vi "main.vi"() -> ()   [LabVIEW 2020]
uses:
  <vilib>/express/express signal manip/GetorSetDDTAttributes/Shared VIs/TimeType.ctl
  5948bca3-3d14-40bf-9fbb-2ba5c3eee3bd.vi
  <vilib>/Analysis/baseanly.llb/Mean (DBL).vi
  faa81322-6883-41b3-8229-1eb533283c0b.vi
  <extravilib>/ChannelInstances/Tag-bool/Read With Abort.vi
  <extravilib>/ChannelInstances/Tag-bool/Write With Abort.vi
  <extravilib>/ChannelInstances/Tag-bool/Instantiate.vi
  <extravilib>/ChannelInstances/Tag-bool/EndpointRead.vi
  <vilib>/express/express signal manip/GetorSetDDTAttributes/Shared VIs/TimeMode Enum to Boolean.vi
  <vilib>/express/express shared/transition.llb/Dynamic To Waveform Array.vi
  <vilib>/express/express signal manip/GetorSetDDTAttributes/Set DDT Attributes/SetT0.vi
  <vilib>/express/express shared/transition.llb/Waveform Array To Dynamic.vi
  <extravilib>/ChannelInstances/Tag-bool/Endpoint.vi
  <vilib>/express/express signal manip/GetorSetDDTAttributes/Set DDT Attributes/Set DDT Properties.xnode
  <extravilib>/ChannelInstances/Tag-bool.lvlib
  <vilib>/ptbypt/NI_PtbyPt.lvlib
  <vilib>/Analysis/NI_AALBase.lvlib
  <vilib>/express/express signal manip/GetorSetDDTAttributes/Shared VIs/GetSetShared.lvlib
panel:
  out "dt":dbl
  in  "?":T1(tab)
  in  "Test Knob":dbl(knob) scale=0.0..10.0
  out "Signal Frequency\n 2":dbl(graph)
  out "Stable RPM measurement?":bool
  in  "Nominal R":dbl
  in  "Nominal Omega":dbl
  in  "Sample rate":dbl=1000.0
  in  "Number of Samples":dbl=5.0
  in  "Voltage Threshold":dbl=0.5
  in  "Number of magnets":dbl=1.0
  out "Omega [RPM]":dbl(knob) scale=0.0..2000.0
  out "Voltage RMS [V]":dbl(knob) scale=0.0..20.0
  out "Power Output [W]":dbl(knob) scale=0.0..20.0
  out "Current RMS [A]":dbl(knob) scale=0.0..20.0
  in  "Button":bool
  out "Signal\nFrequency (Hz)":dbl
  in  "?":bool
  in  "Button 2":bool
  out "Python Error Status":errorcluster
  in  "Filename":path=path "C:/Users/johan/OneDrive - Estudiantes ITCR/TEC/ProyectodeGraduacion/LabEolicaControl/rawdata.txt"
  out "Voltage Sensor":dynamicdata(graph)
  out "Current Sensor":dynamicdata(graph)
  out "Hall sensor\n 2":dynamicdata(graph)
  out "Hall sensor":dynamicdata(graph)
  # "Lab Setup"
  # "Post Processing"
  # "Data Monitoring"
  # "Real Time Analysis variables"
  # "Measurement Point"
  # "File I/O"
  # "About:"
  # "Software Requirements:"
  # "This measuring system was designed for data acquisition of \npower, angular speed, and resistance data for small scale HAWT \nand possibly VAWT. These turbines are being researched and \ndeveloped at LIENE (Laboratorio de Investigación en Energía Eólica) \nat ITCR. \n\nThis software acquires data and performs post processing to obtain \npower graphs and surfaces and data tables for further analysis. It uses \nLabView for DAQ and integrated Python scripts to post process and \ngraph data."
  # "Python 3.6 with the following packages:\n-- NumPy\n-- Plotly"
  # "Programmer:"
  # "This software was designed and programmed by: \n-- Johansell Villalobos Cubillo: \n         Engineering Physics student"
  # "DAQ Equipment: NI-USB-6000"
  # "The equipment pinout diagram is shown below and the pins are used as follows: \n\nAl 0 -- Hall effect sensor\nAl 1 -- ACS712 10A current sensor\nAl 2 -- Voltage sensor\nAl GND -- common ground"
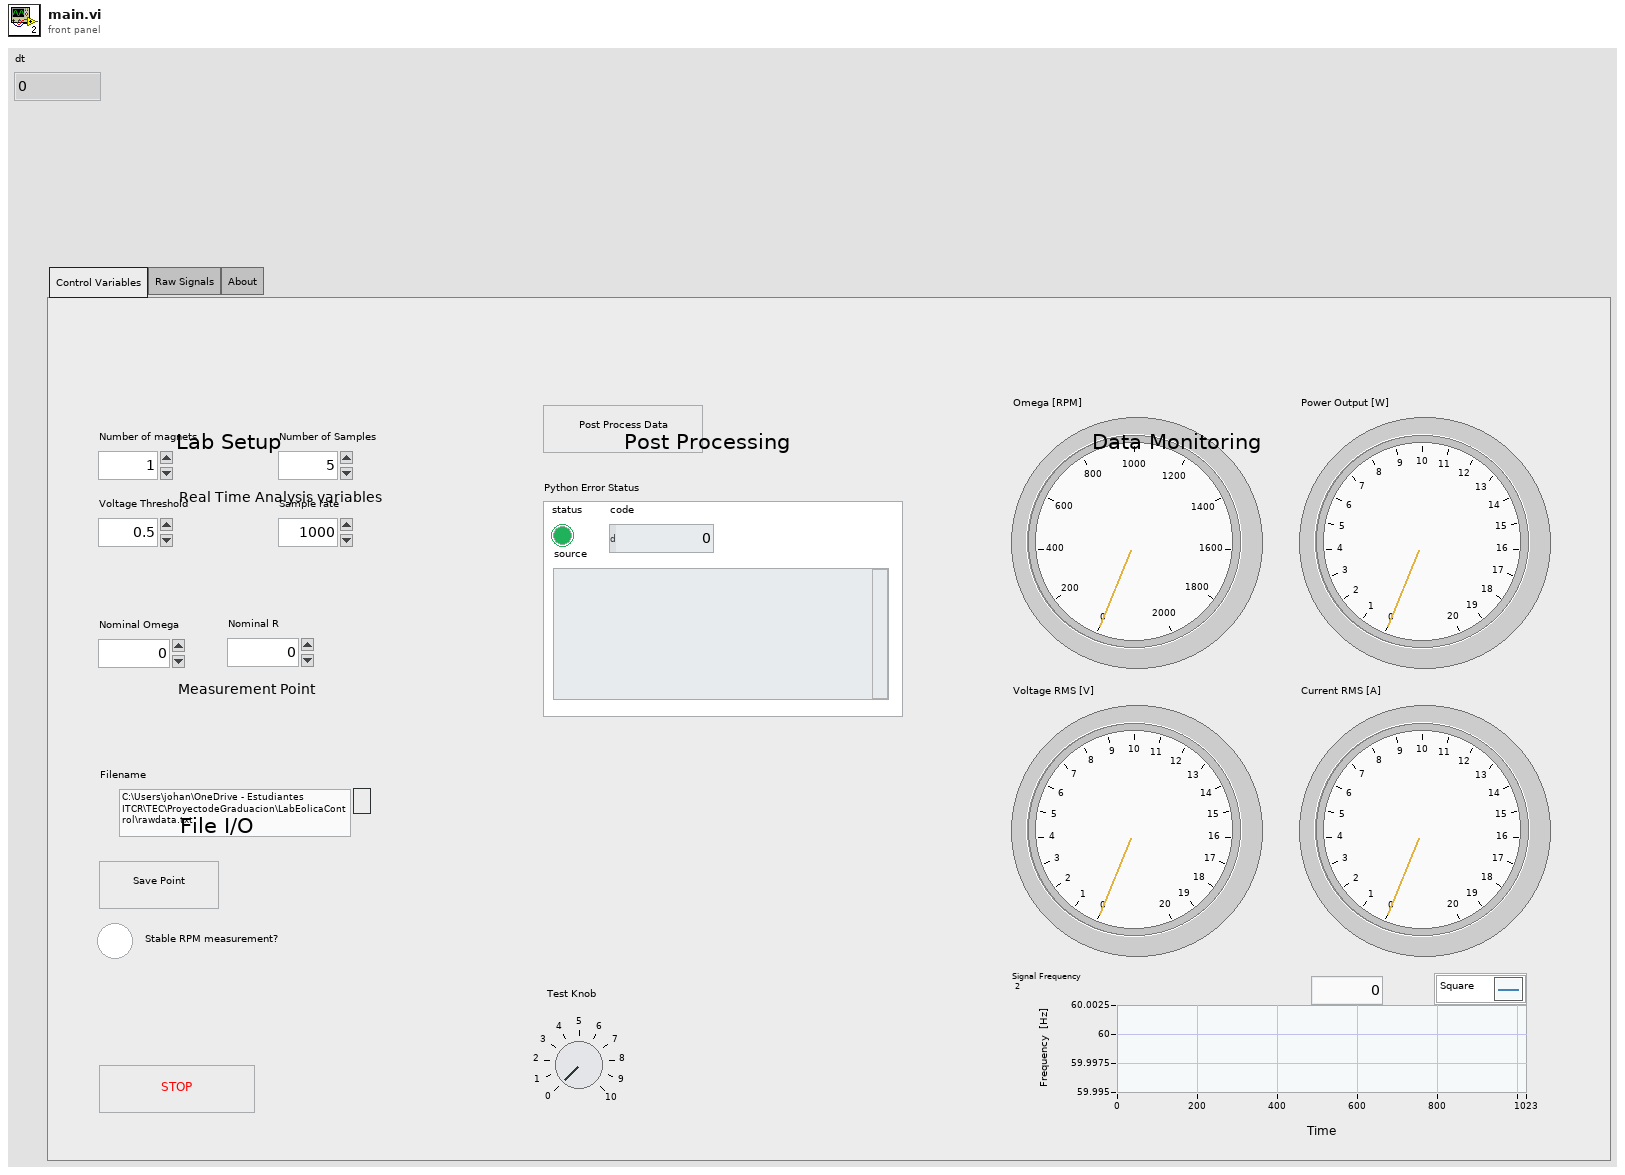
[diagram p1: front panel]
types:
  T1 = enum32{"Control Variables", "Raw Signals", "About"}
  T2 = typedef "Tag-bool.lvlib/))Channel.ctl" = refnum<queue>
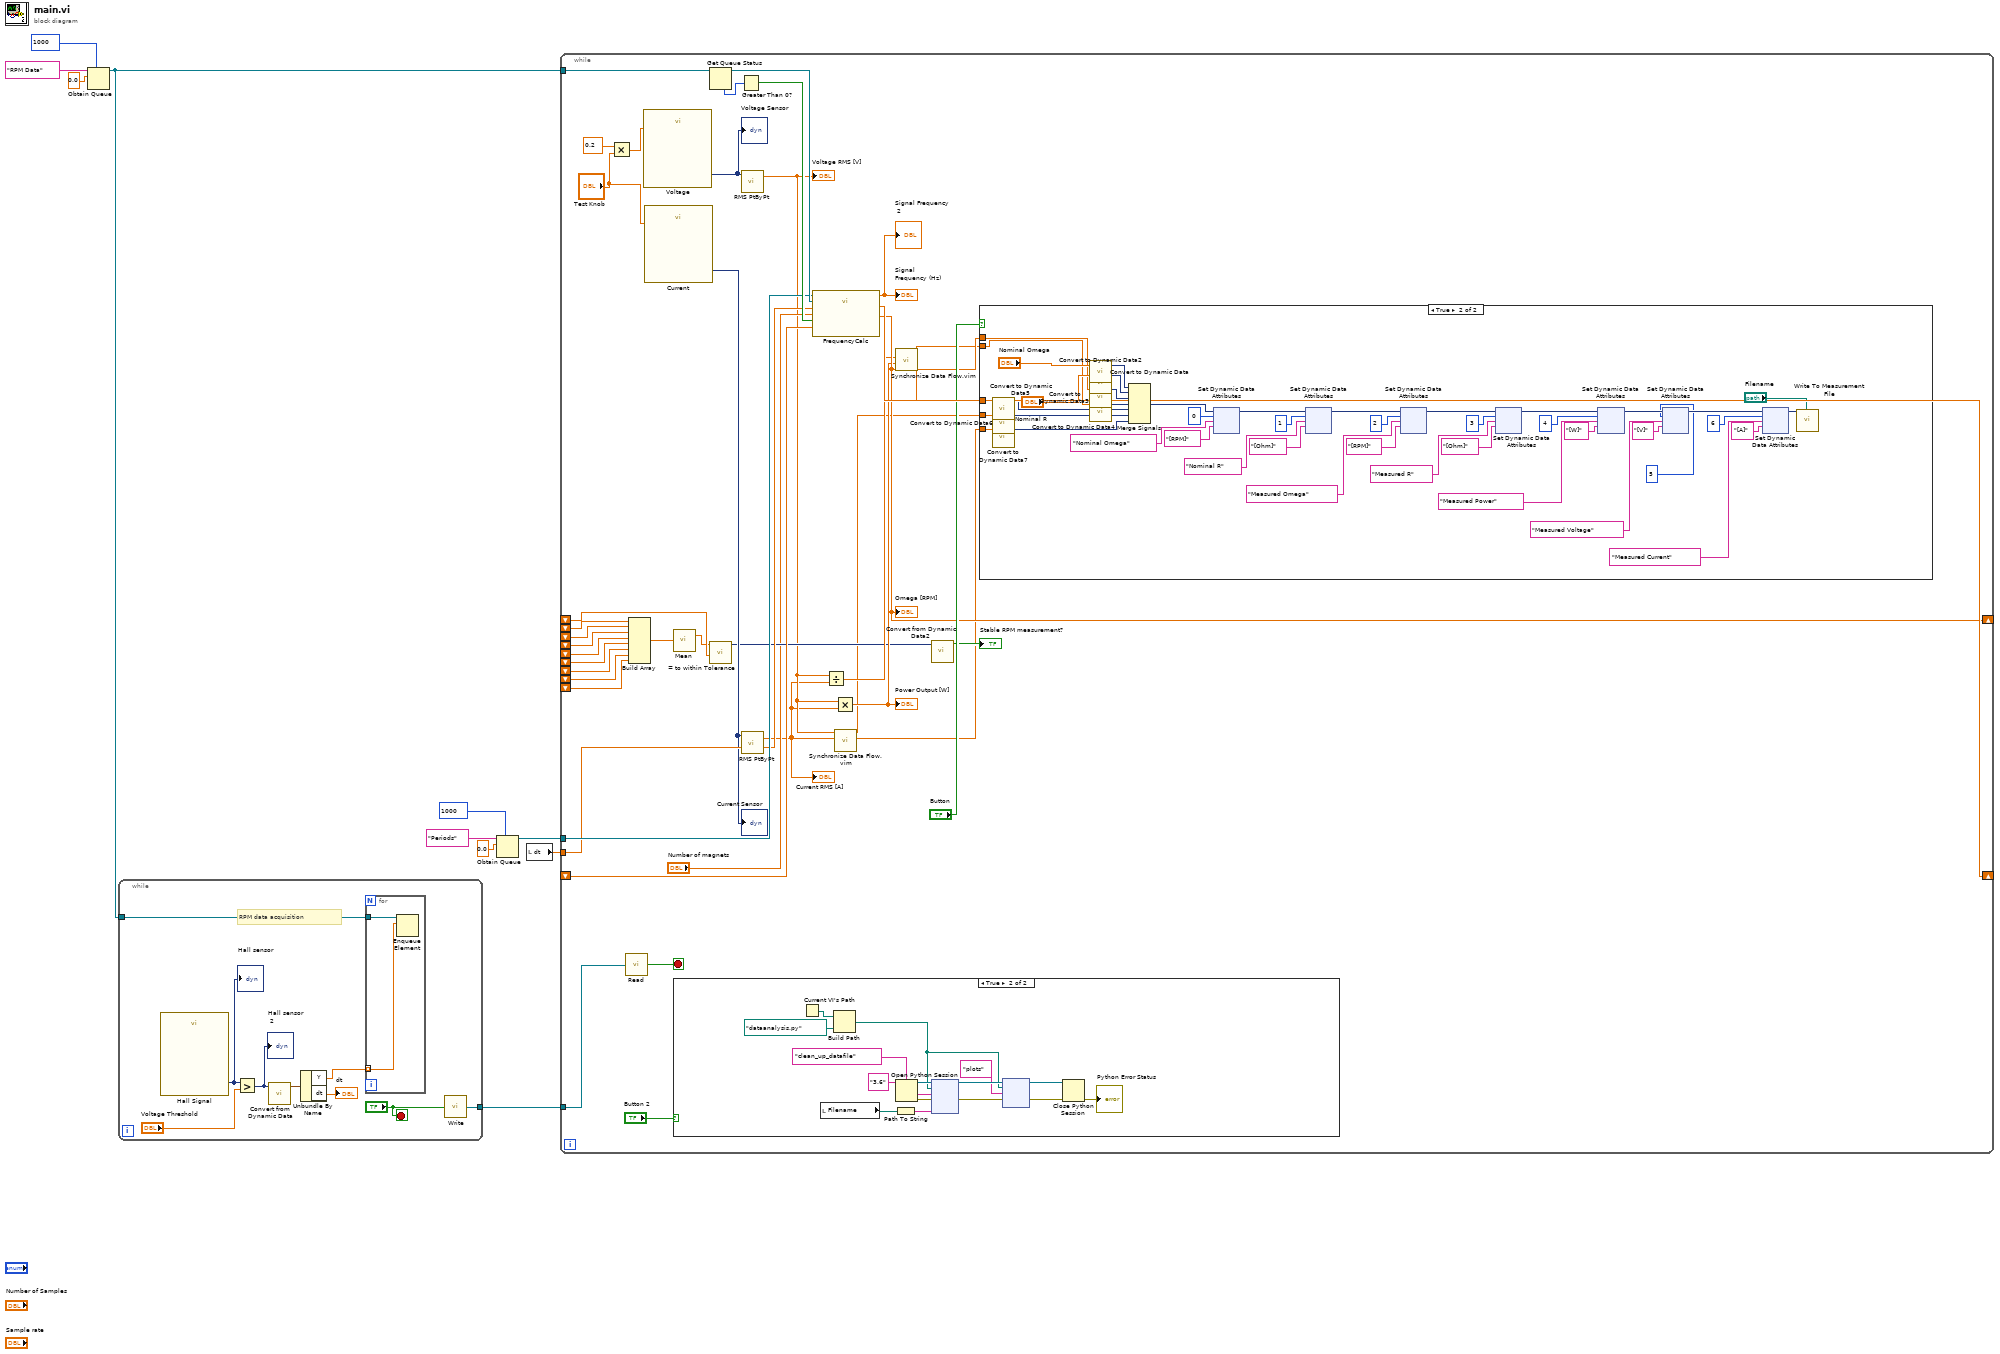
[diagram p0: block diagram]
diagram:
  n1 = Obtain Queue(max queue size (-1, unlimited)=1000 ("max queue size\n(-1, unlimited)"), name (unnamed)="RPM Data" ("name\n(unnamed)"), element data type=0.0 ("data type\n(double)")) -> (queue out=w5:refnum<queue>)  [unwired: 2 in, 2 out]
  n2 = while {
    tunnel: w5 -> [w17]
    tunnel: [w13] -> w7
    stop <- "?" stop-if-true
    # "RPM data acquisition"
    n3 = call "Hall Signal"() -> ("Square"=w15:dynamicdata)  [unwired: 14 in, 1 out]
    "Hall sensor" <- w15
    n4 = Greater?(x=w15, y="Voltage Threshold") -> (0:w14:dynamicdata)
    "Hall sensor\n 2" <- w14
    n5 = call "Convert from Dynamic Data"("Dynamic Data Type"=w14) -> ("Waveform"=w19:waveform(dbl))  [unwired: 3 in]
    n6 = Unbundle By Name(w19) -> ("Y"=w18:dbl[], "dt"=→"dt":dbl)
    n7 = for {
      tunnel: w18 -> [w21] mode=indexing
      tunnel: w17 -> [w20]
      n8 = Enqueue Element(queue=w20, element=w21) -> ()  [unwired: 2 in, 3 out]
    }
    n9 = call <extravilib>:"Write.vi"("element"="?") -> ("channel"=w13:T2)  [unwired: 1 out]
  }
  n10 = Obtain Queue(max queue size (-1, unlimited)=1000 ("max queue size\n(-1, unlimited)"), name (unnamed)="Periods" ("name\n(unnamed)"), element data type=0.0 ("data type\n(double)")) -> (queue out=w1:refnum<queue>)  [unwired: 2 in, 2 out]
  n11 = local read "dt"() -> (w6:dbl)
  n12 = while {
    tunnel: w5 -> [w62]
    tunnel: w1 -> [w59]
    shift-right: [w57] -> _
    shift-left: _ -> [w58]
    tunnel: w6 -> [w54]
    tunnel: w7 -> [w55]
    shift-right: [w50] -> _
    shift-left: _ -> [w44]
    shift-left: _ -> [w45]
    shift-left: _ -> [w46]
    shift-left: _ -> [w47]
    shift-left: _ -> [w42]
    shift-left: _ -> [w33]
    shift-left: _ -> [w32]
    shift-left: _ -> [w31]
    shift-left: _ -> [w30]
    stop <- w56 stop-if-true
    n13 = Multiply(x=0.2, y="Test Knob") -> (x*y=w24:dbl)
    n14 = call <extravilib>:"Read.vi"("channel"=w55) -> ("element"=w56:bool)  [unwired: 1 in, 1 out]
    n15 = Build Array(w47, w46, w45, w44, w33, w32, w31, w30) -> (w43:dbl[])
    n16 = call "Voltage"("Amplitude"=w24) -> ("Sine"=w52:dynamicdata)  [unwired: 13 in, 1 out]
    "Voltage Sensor" <- w52
    n17 = call "Current"("Amplitude"="Test Knob") -> ("Sine"=w53:dynamicdata)  [unwired: 13 in, 1 out]
    "Current Sensor" <- w53
    n18 = call-poly <vilib>:"Mean.vi"("X"=w43) -> ("mean"=w41:dbl)  [unwired: 1 out]
    n19 = case shown="True" "Button 2" {
      frame False {
      }
      frame True {
        n20 = Current VI's Path() -> (path=w71:path)
        n21 = local read "Filename"() -> (w74:path)
        n22 = Build Path(base path=w71, name or relative path=path "dataanalysis.py") -> (appended path=w68:path)
        n23 = Path To String(path=w74) -> (string=w75:string)
        n24 = Open Python Session(python version="3.6" ("Python version")) -> (session out=w76:refnum<k35>, error out=w77:errorcluster)  [unwired: 2 in]
        n25 = node(w76, w68, "clean_up_datafile" ("function name"), w77, w75) -> (w69:refnum<k35>, w66:errorcluster)  [unwired: 3 in, 2 out]
        n26 = node(w69, w68, "plots" ("function name"), w66) -> (w64:refnum<k35>, w65:errorcluster)  [unwired: 2 in, 2 out]
        n27 = Close Python Session(session in=w64, error in=w65) -> (11:→"Python Error Status":errorcluster)
      }
    }
    n28 = Get Queue Status(queue=w62) -> (queue out=w60:refnum<queue>, # elements in queue=w63:i32)  [unwired: 2 in, 6 out]
    n29 = call "= to within Tolerance"("Constant Value to Compare Against"=w42, "Operand 1"=w41) -> ("Result"=w40:dynamicdata)  [unwired: 8 in, 1 out]
    n30 = Greater Than 0?(x=w63) -> (x > 0?=w61:bool)
    n31 = call <vilib>:"RMS PtByPt.vi"("x"=w52) -> ("rms value"=w28:dbl)  [unwired: 3 in, 1 out]
    "Voltage RMS [V]" <- w28
    n32 = call <vilib>:"RMS PtByPt.vi"("x"=w53) -> ("rms value"=w27:dbl)  [unwired: 3 in, 1 out]
    "Current RMS [A]" <- w27
    n33 = call "FrequencyCalc.vi"("Checkbox"=w61, "Number of teeth in gear"="Number of magnets", "Period\n(s) in"=w58, "dt"=w54, "queue in"=w60, "Queue in"=w59) -> ("Omega [RPM]"=w50:dbl, "Period\n(s) out"=w57:dbl, "Signal Frequency (Hz)"=→"Signal\nFrequency (Hz)" →"Signal Frequency\n 2":dbl)  [unwired: 2 in, 1 out]
    "Omega [RPM]" <- w50
    n34 = Divide(x=w28, y=w27) -> (x/y=w49:dbl)
    n35 = Multiply(x=w28, y=w27) -> (x*y=w48:dbl)
    "Power Output [W]" <- w48
    n36 = call "Synchronize Data Flow.vim"("input 2"=w27, "input 1"=w28) -> ("output 2"=w25:dbl, "output 1"=w26:dbl)  [unwired: 2 in, 2 out]
    n37 = call "Synchronize Data Flow.vim"("input 4"=w50, "input 3"=w48, "input 2"=w49) -> ("output 4"=w38:dbl, "output 3"=w36:dbl, "output 2"=w37:dbl)  [unwired: 1 in, 1 out]
    n38 = call "Convert from Dynamic Data2"("Dynamic Data Type"=w40) -> ("Scalar"=→"Stable RPM measurement?":bool)  [unwired: 3 in]
    n39 = case shown="True" "Button" {
      tunnel: w38 -> [_ w117]
      tunnel: w37 -> [_ w118]
      tunnel: w36 -> [_ w113]
      tunnel: w26 -> [_ w91]
      tunnel: w25 -> [_ w90]
      frame False {
      }
      frame True {
        n40 = call "Convert to Dynamic Data5"("Double"=w113) -> ("Dynamic Data Type"=w114:dynamicdata)  [unwired: 3 in]
        n41 = call "Convert to Dynamic Data6"("Double"=w91) -> ("Dynamic Data Type"=w89:dynamicdata)  [unwired: 3 in]
        n42 = call "Convert to Dynamic Data7"("Double"=w90) -> ("Dynamic Data Type"=w88:dynamicdata)  [unwired: 3 in]
        n43 = call "Convert to Dynamic Data"("Double"="Nominal Omega") -> ("Dynamic Data Type"=w120:dynamicdata)  [unwired: 3 in]
        n44 = call "Convert to Dynamic Data2"("Double"="Nominal R") -> ("Dynamic Data Type"=w119:dynamicdata)  [unwired: 3 in]
        n45 = call "Convert to Dynamic Data3"("Double"=w117) -> ("Dynamic Data Type"=w116:dynamicdata)  [unwired: 3 in]
        n46 = call "Convert to Dynamic Data4"("Double"=w118) -> ("Dynamic Data Type"=w115:dynamicdata)  [unwired: 3 in]
        n47 = Merge Signals(w120, w119, w116, w115, w114, w89, w88) -> (w112:dynamicdata)
        n48 = xnode ("Set Dynamic Data Attributes")("Signals In"=w112, "Signal Index"=0, "Signal Name"="Nominal Omega", "Unit"="[RPM]") -> ("Signals Out"=w105:dynamicdata)  [unwired: 3 in, 1 out]
        n49 = xnode ("Set Dynamic Data Attributes")("Signals In"=w105, "Signal Index"=1, "Signal Name"="Nominal R", "Unit"="[Ohm]") -> ("Signals Out"=w101:dynamicdata)  [unwired: 3 in, 1 out]
        n50 = xnode ("Set Dynamic Data Attributes")("Signals In"=w101, "Signal Index"=2, "Signal Name"="Measured Omega", "Unit"="[RPM]") -> ("Signals Out"=w97:dynamicdata)  [unwired: 3 in, 1 out]
        n51 = xnode ("Set Dynamic Data Attributes")("Signals In"=w97, "Signal Index"=3, "Signal Name"="Measured R", "Unit"="[Ohm]") -> ("Signals Out"=w93:dynamicdata)  [unwired: 3 in, 1 out]
        n52 = xnode ("Set Dynamic Data Attributes")("Signals In"=w93, "Signal Index"=4, "Signal Name"="Measured Power", "Unit"="[W]") -> ("Signals Out"=w81:dynamicdata)  [unwired: 3 in, 1 out]
        n53 = xnode ("Set Dynamic Data Attributes")("Signals In"=w81, "Signal Index"=5, "Signal Name"="Measured Voltage", "Unit"="[V]") -> ("Signals Out"=w83:dynamicdata)  [unwired: 3 in, 1 out]
        n54 = xnode ("Set Dynamic Data Attributes")("Signals In"=w83, "Signal Index"=6, "Signal Name"="Measured Current", "Unit"="[A]") -> ("Signals Out"=w80:dynamicdata)  [unwired: 3 in, 1 out]
        n55 = call "Write To Measurement File"("Signals"=w80, "Filename"="Filename") -> ()  [unwired: 15 in, 3 out]
      }
    }
  }
